vi "Register Events.vi"(0 "Display State In":T2={"WebView2 Ref"=refnum, "event callback refnum"=refnum, "Events"={"Navigation Complete Event"=refnum, "Source Changed Event"=refnum, "Document Title Changed Event"=refnum, "Status Bar Text Changed"=refnum, "Web Message Received"=refnum, "Window Close Requested"=refnum}, "Paths"={"Webview2 Native"=path "C:/Users/kleins/Desktop/webview2/microsoft.web.webview2.1.0.1370.28/build/native", "Edge Application"=path "", "User Data"=path ""}}, 9 "Container State":T4, 11 "error in (no error)":errorcluster) -> (4 "Display State Out":T2={"WebView2 Ref"=refnum, "event callback refnum"=refnum, "Events"={"Navigation Complete Event"=refnum, "Source Changed Event"=refnum, "Document Title Changed Event"=refnum, "Status Bar Text Changed"=refnum, "Web Message Received"=refnum, "Window Close Requested"=refnum}, "Paths"={"Webview2 Native"=path "C:/Users/kleins/Desktop/webview2/microsoft.web.webview2.1.0.1370.28/build/native", "Edge Application"=path "", "User Data"=path ""}}, 6 "Events":T1, 15 "error out":errorcluster)   [LabVIEW 2020, in "WebView2 Control.xctl"]
uses:
  WebView2 Control.xctl
  <vilib>/_xctls/Container State.ctl
  State.ctl
  E:/Labview/LV 2020/Libs/LV-WebView2/microsoft.web.webview2/lib/net45/Microsoft.Web.WebView2.WinForms.dll
  microsoft.web.webview2/lib/net45/Microsoft.Web.WebView2.WinForms.dll
  Paths.ctl
  _Raise Nav Complete Event.vi
  _Raise Navigation Starting Event.vi
  _Raise Source Changed Event.vi
  _Raise Document Title Changed.vi
  _Raise StatusBarTextChanged.vi
  _Raise WebMessageReceived.vi
  _Raise WindowCloseRequested.vi
  E:/Labview/LV 2020/Libs/LV-WebView2/microsoft.web.webview2/lib/net45/Microsoft.Web.WebView2.Core.dll
  microsoft.web.webview2/lib/net45/Microsoft.Web.WebView2.Core.dll
  <vilib>/_xctls/XControlSupport.lvlib
panel:
  # "Add Controls & Indicators that form the parameters of the method here. Hook them to the connector pane. Do not delete the controls & indicators that are already hooked to the connector pane.\n \nTo setup the parameters  for this method, right click on this item in the Project Tree & select \"Configure Method...\"."
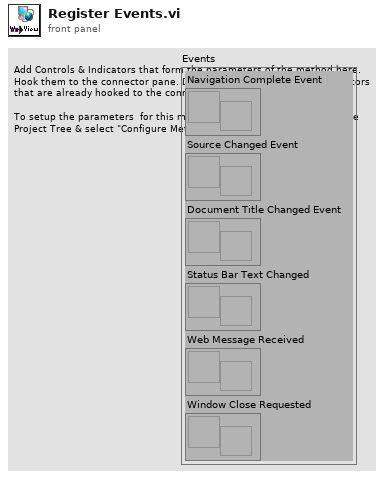
[diagram p1: front panel]
types:
  T1 = cluster{"Navigation Complete Event":refnum<user-event>, "Source Changed Event":refnum<user-event>, "Document Title Changed Event":refnum<user-event>, "Status Bar Text Changed":refnum<user-event>, "Web Message Received":refnum<user-event>, "Window Close Requested":refnum<user-event>}
  T2 = typedef "WebView2 Control.xctl/State.ctl" = cluster{"WebView2 Ref":refnum<data-value>, "event callback refnum":refnum<k27>, "Events":cluster{"Navigation Complete Event":refnum<user-event>, "Source Changed Event":refnum<user-event>, "Document Title Changed Event":refnum<user-event>, "Status Bar Text Changed":refnum<user-event>, "Web Message Received":refnum<user-event>, "Window Close Requested":refnum<user-event>}, "Paths":T3}
  T3 = typedef "WebView2 Control.xctl/Paths.ctl" = cluster{"Webview2 Native":path, "Edge Application":path, "User Data":path}
  T4 = typedef "XControlSupport.lvlib/Container State.ctl" = cluster{"Indicator?":bool, "Run Mode?":bool, " Refnum":refnum<vi>}
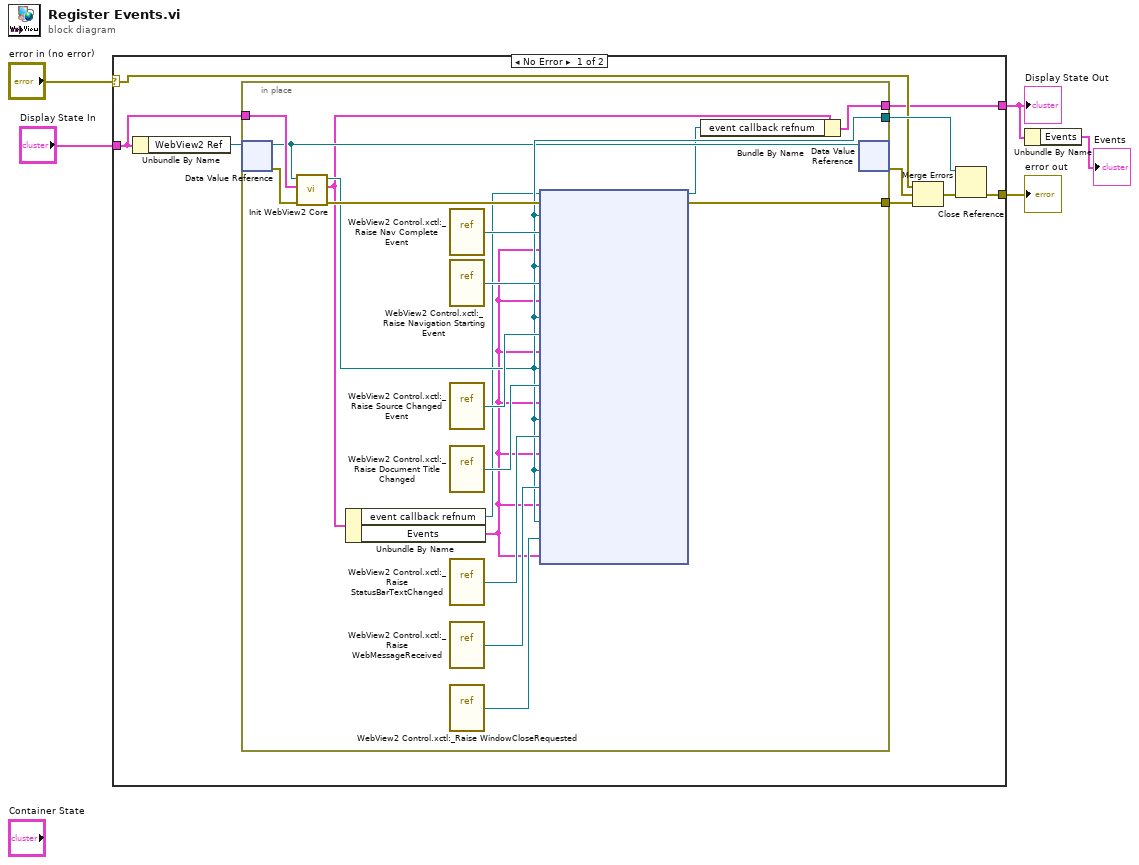
[diagram p0: block diagram]
diagram:
  n1 = case shown="No Error" "error in (no error)" {
    selector: "error in (no error)" -> [w7 w34]
    tunnel: [w6 w33] -> w2
    tunnel: "Display State In" -> [w13 w33]
    tunnel: [w12 w34] -> w4
    frame No Error {
      n2 = Unbundle By Name(w13) -> ("WebView2 Ref"=w14:refnum<data-value>)
      n3 = in-place {
        in-place-border: [w32] -> w10
        in-place-border: [w23] -> w8
        in-place-border: w13 -> [w22]
        in-place-border: [w15] -> w6
        n4 = in-place-dvr #1(w14) -> (w21:refnum<k24>, w20:errorcluster)
        n5 = call "Init WebView2 Core.vi"("error in (no error)"=w20, "Display State In"=w22, ".NET Refnum in"=w21) -> ("error out"=w24:errorcluster, "Display State In 2"=w19:T2, ".NET Refnum out"=w23:refnum<k24>)  [unwired: 6 in]
        n6 = Unbundle By Name(w19) -> ("event callback refnum"=w17:refnum<k27>, "Events"=w18:T1)
        n7 = vi-ref "WebView2 Control.xctl:_Raise Nav Complete Event.vi"() -> ("vi reference"=w25:refnum<vi>)
        n8 = vi-ref "WebView2 Control.xctl:_Raise Navigation Starting Event.vi"() -> ("vi reference"=w31:refnum<vi>)
        n9 = vi-ref "WebView2 Control.xctl:_Raise Source Changed Event.vi"() -> ("vi reference"=w30:refnum<vi>)
        n10 = vi-ref "WebView2 Control.xctl:_Raise Document Title Changed.vi"() -> ("vi reference"=w29:refnum<vi>)
        n11 = vi-ref "WebView2 Control.xctl:_Raise StatusBarTextChanged.vi"() -> ("vi reference"=w28:refnum<vi>)
        n12 = vi-ref "WebView2 Control.xctl:_Raise WebMessageReceived.vi"() -> ("vi reference"=w27:refnum<vi>)
        n13 = vi-ref "WebView2 Control.xctl:_Raise WindowCloseRequested.vi"() -> ("vi reference"=w26:refnum<vi>)
        n14 = node(w17, w24, w23, w25, w18, w23, w31, w18, w23, w30, w18, w23, w29, w18, w23, w28, w18, w23, w27, w18, w23, w26, w18) -> (w16:refnum<k27>, w32:errorcluster)
        n15 = Bundle By Name(cluster=w19, "event callback refnum"=w16) -> (w15:T2)
        n16 = in-place-dvr #1(w21) -> (w11:errorcluster)  [unwired: 1 out]
      }
      n17 = Merge Errors(w7, w11, w10) -> (w9:errorcluster)
      n18 = Close Reference(reference=w8, error in (no error)=w9) -> (error out=w12:errorcluster)
    }
    frame Error {
    }
  }
  "Display State Out" <- w2
  "error out" <- w4
  n19 = Unbundle By Name(w2) -> ("Events"=→"Events":T1)
